vi "Instrument_Write&Read_HIPOT.vi"(8 "Error In":errorcluster, 10 "PORT":string, 11 "Limit":string) -> (0 "error out":errorcluster, 2 "Result":bool, 3 "Data":string)   [LabVIEW 2013]
uses:
  MainProgram/Control/Buffer.vi
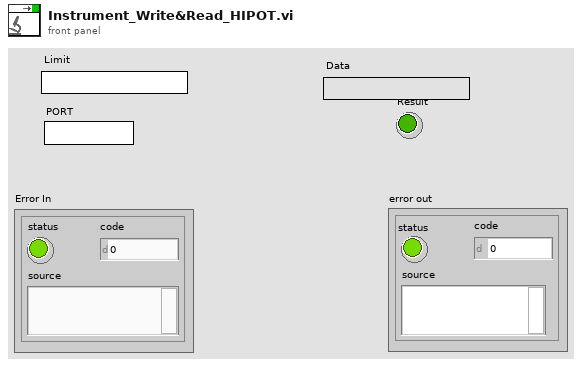
[diagram p1: front panel]
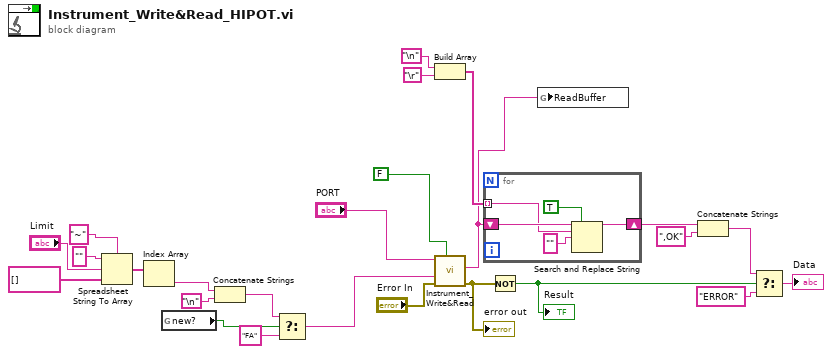
[diagram p0: block diagram]
diagram:
  n1 = Spreadsheet String To Array(delimiter (Tab)="~", format string="", spreadsheet string="Limit", array type (2D Dbl)=string[] []) -> (array=w19:string[])
  n2 = Index Array(array=w19) -> (element=w7:string)  [unwired: 1 in]
  n3 = global read "Buffer.vi" "new?"() -> (w4:bool)
  n4 = Concatenate Strings(w7, "\n") -> (w3:string)
  n5 = Select(t=w3, s=w4, f="FA") -> (s? t:f=w2:string)
  n6 = Build Array("\n", "\r") -> (w11:string[])
  n7 = call "Instrument_Write&Read.vi"("Read?"=FALSE, "Error In"="Error In", "CMD"=w2, "PORT"="PORT") -> ("Error Out"=w16:errorcluster, "read buffer"=w5:string)  [unwired: 6 in]
  "error out" <- w16
  n8 = for {
    tunnel: w11 -> [w27] mode=indexing
    shift-right: [w26] -> w10
    shift-left: w5 -> [w30]
    n9 = Search and Replace String(replace all?=TRUE ("replace all? (F)"), input string=w30, search string=w27, replace string="" ("replace string (\"\")")) -> (result string=w26:string)  [unwired: 4 in, 3 out]
  }
  n10 = Not(x=w16) -> (.not. x?=w23:bool)
  "Result" <- w23
  n11 = global write "Buffer.vi" "ReadBuffer"(w5) -> ()
  n12 = Concatenate Strings(w10, ",OK") -> (w14:string)
  n13 = Select(t=w14, s=w23, f="ERROR") -> (s? t:f=→"Data":string)
